vi "02_write_file_errorhadling.vi"() -> ()   [LabVIEW 2017]
panel:
  in  "stop":bool
  in  "file path (use dialog)":path
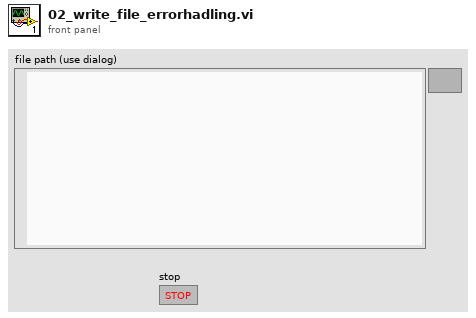
[diagram p1: front panel]
types:
  T1 = enum16{"open", "replace", "create", "open or create", "replace or create", "replace or create with confirmation"}
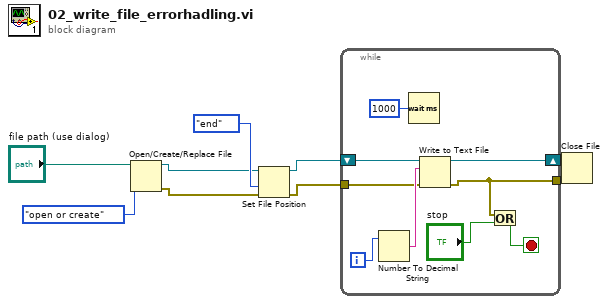
[diagram p0: block diagram]
diagram:
  n1 = Open/Create/Replace File(file path (use dialog)="file path (use dialog)", operation (0:open)=T1."open or create") -> (refnum out=w5:refnum<file>, error out=w3:errorcluster)  [unwired: 4 in, 1 out]
  n2 = Set File Position(refnum=w5, from (0:start)=enum16{"start", "end", "current"}."end", error in=w3) -> (refnum out=w4:refnum<file>, error out=w2:errorcluster)  [unwired: 1 in]
  n3 = while {
    shift-right: [w18] -> w7
    shift-left: w4 -> [w17]
    tunnel: w2 -> [w13]
    tunnel: [w12] -> w1
    i -> [w15]
    stop <- w10 stop-if-true
    n4 = Number To Decimal String(number=w15) -> (decimal integer string=w16:string)  [unwired: 1 in]
    n5 = Wait (ms)(milliseconds to wait=u32 1000) -> ()  [unwired: 1 out]
    n6 = Write to Text File(file (use dialog)=w17, text=w16, error in=w13) -> (refnum out=w18:refnum<file>, error out=w12:errorcluster)  [unwired: 1 in, 1 out]
    n7 = Or(x=w12, y="stop") -> (x .or. y?=w10:bool)
  }
  n8 = Close File(refnum=w7, error in=w1) -> ()  [unwired: 2 out]
